vi "首页设置全局变量.vi"() -> ()   [LabVIEW 2016]
panel:
  in  "磷酸盐":bool caption="氨氮禁用"
  in  "CODCr":bool caption="氨氮禁用"
  in  "ORP":bool caption="氨氮禁用"
  in  "硫化物":bool caption="氨氮禁用"
  in  "亚硝氮":bool caption="氨氮禁用"
  in  "硝氮":bool caption="氨氮禁用"
  in  "藻密度":bool caption="氨氮禁用"
  in  "叶绿素a":bool caption="氨氮禁用"
  in  "湿度":bool caption="氨氮禁用"
  in  "室温":bool caption="氨氮禁用"
  in  "电压":bool caption="氨氮禁用"
  in  "CODMn":bool=TRUE caption="氨氮禁用"
  in  "总氮":bool=TRUE caption="氨氮禁用"
  in  "总磷":bool=TRUE caption="氨氮禁用"
  in  "氨氮":bool=TRUE caption="氨氮禁用"
  in  "Turb":bool=TRUE caption="氨氮禁用"
  in  "Cond":bool=TRUE caption="氨氮禁用"
  in  "DO":bool=TRUE caption="氨氮禁用"
  in  "pH":bool=TRUE caption="氨氮禁用"
  in  "水温":bool=TRUE caption="氨氮禁用"
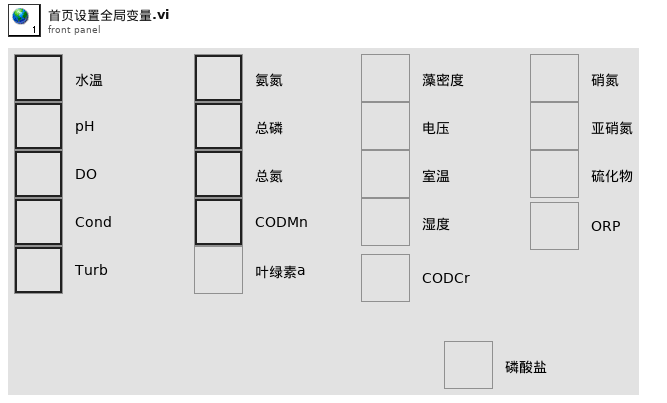
[diagram p1: front panel]
diagram:
